vi "WS1050_36DUT_Cycle SubVI.vi"(8 "error out":errorcluster, 9 "Number of Cycle (X1000)":dbl, 10 "Post CMd Delay":dbl[](array[numeric])=[1.2e-05, 5.4e-05, 1.8e-05] min=0.0 max=0.5 format="%#.0p s", 11 "Command":string[](array[string])=["0702013B3B3B", "070201000000", "0702013B0000"]) -> (0 "Error Out":errorcluster, 3 "Cycle Count":u64 min=1 max=4 step=1)   [LabVIEW 2012]
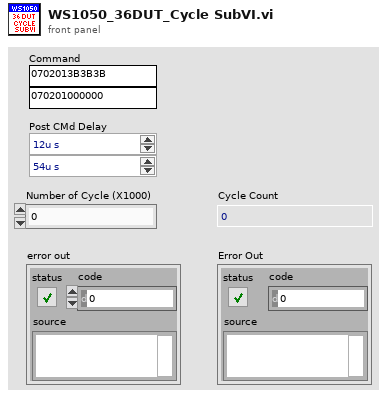
[diagram p1: front panel]
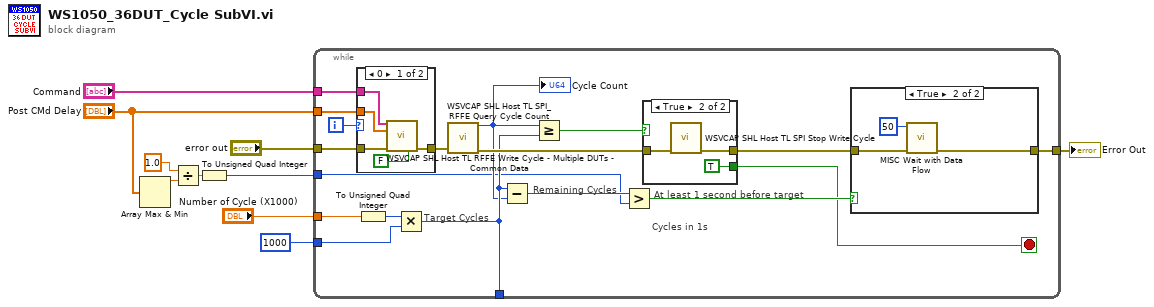
[diagram p0: block diagram]
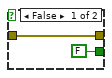
[diagram p4: hidden frame]
diagram:
  n1 = Array Max & Min(array="Post CMd Delay") -> (max value=w5:dbl)  [unwired: 3 out]
  n2 = Divide(x=1.0, y=w5) -> (x/y=w6:dbl)
  n3 = To Unsigned Quad Integer(1:w6) -> (0:w3:u64)
  n4 = while {
    tunnel: "Number of Cycle (X1000)" -> [w28]
    tunnel: [w18] -> w9
    tunnel: "error out" -> [w26]
    tunnel: [w17] -> _
    tunnel: "Command" -> [w25]
    tunnel: "Post CMd Delay" -> [w24]
    tunnel: w3 -> [w14]
    tunnel: u64 1000 ("y") -> [w12]
    i -> [w23]
    stop <- w11 stop-if-true
    # "At least 1 second before target"
    # "Remaining Cycles"
    # "Target Cycles"
    # "Cycles in 1s"
    n5 = case shown="0" w23 {
      tunnel: [w36 w38] -> w20
      tunnel: w26 -> [w37 w38]
      tunnel: w25 -> [w35 _]
      tunnel: w24 -> [w34 _]
      frame 0 {
        n6 = call "WSVCAP SHL Host TL RFFE Write Cycle - Multiple DUTs - Common Data.vi"("Data Out (Cycle Commands)"=w35, "Post Command Delay"=w34, "error in"=w37, "Log (T)"=FALSE) -> ("error out"=w36:errorcluster)  [unwired: 11 in]
      }
      frame 1, Default {
      }
    }
    n7 = To Unsigned Quad Integer(1:w28) -> (0:w27:u64)
    n8 = Multiply(x=w27, y=w12) -> (x*y=w17:u64)
    n9 = call "WSVCAP SHL Host TL SPI_RFFE Query Cycle Count.vi"("error in"=w20) -> ("Cycle Count"=w16:u64, "error out"=w22:errorcluster)  [unwired: 13 in]
    "Cycle Count" <- w16
    n10 = Subtract(x=w17, y=w16) -> (x-y=w15:u64)
    n11 = Greater Or Equal?(x=w16, y=w17) -> (x >= y?=w21:bool)
    n12 = Greater?(x=w15, y=w14) -> (0:w13:bool)
    n13 = case shown="True" w21 {
      tunnel: [w40 w43] -> w19
      tunnel: w22 -> [w40 w42]
      tunnel: [FALSE TRUE] -> w11
      frame False {
      }
      frame True {
        n14 = call "WSVCAP SHL Host TL SPI Stop Write Cycle.vi"("error in"=w42) -> ("error out"=w43:errorcluster)  [unwired: 14 in]
      }
    }
    n15 = case shown="True" w13 {
      tunnel: w19 -> [w29 w32]
      tunnel: [w29 w31] -> w18
      frame False {
      }
      frame True {
        n16 = call "MISC Wait with Data Flow.vi"("Error In (no error)"=w32, "Wait Time (500ms)"=u32 50) -> ("Error Out"=w31:errorcluster)  [unwired: 7 in, 2 out]
      }
    }
  }
  "Error Out" <- w9
